vi "demo04_medCal.vi"() -> ()   [LabVIEW 2017]
panel:
  out "过程显示":string
  out "结果":string
  out "输入  2":string
  out "输入  1":string
  out "输入 临时值":string
  out "操作 临时值":string
  in  "操作 等于":bool
  in  "操作 清除":bool
  in  "操作 /":bool
  in  "操作 *":bool
  in  "操作 -":bool
  in  "操作 +":bool
  in  "小数点":bool
  in  "数字 0":bool
  in  "+/-":bool
  in  "数字 9":bool
  in  "数字 8":bool
  in  "数字 7":bool
  in  "数字 6":bool
  in  "数字 5":bool
  in  "数字 4":bool
  in  "数字 3":bool
  in  "数字 2":bool
  in  "数字 1":bool
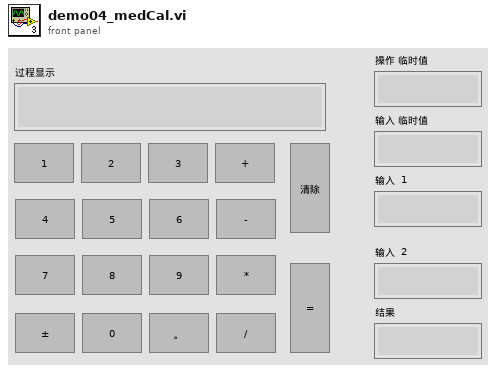
[diagram p1: front panel]
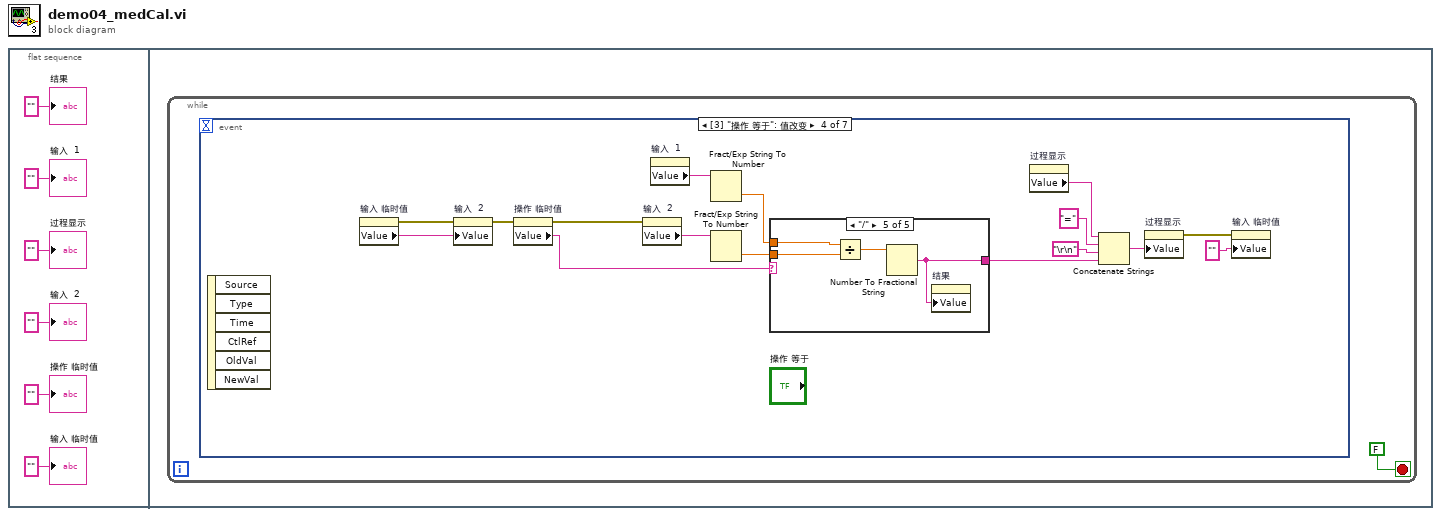
[diagram p0: block diagram]
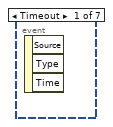
[diagram p2: hidden frame]
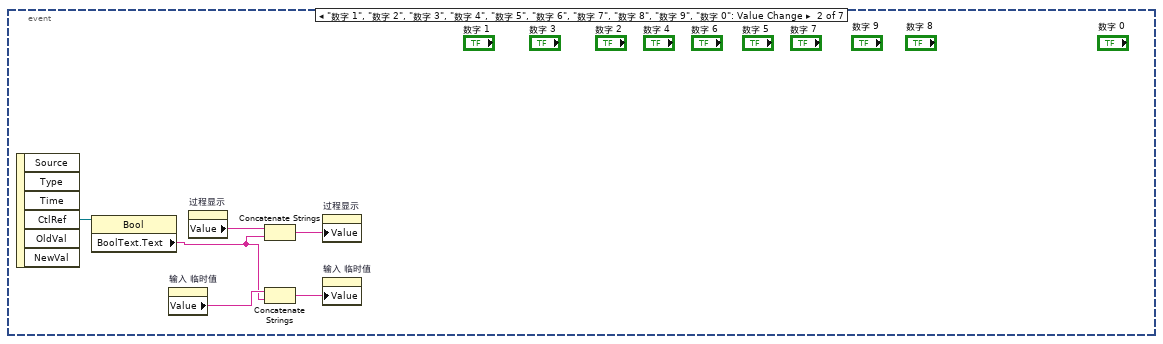
[diagram p3: hidden frame]
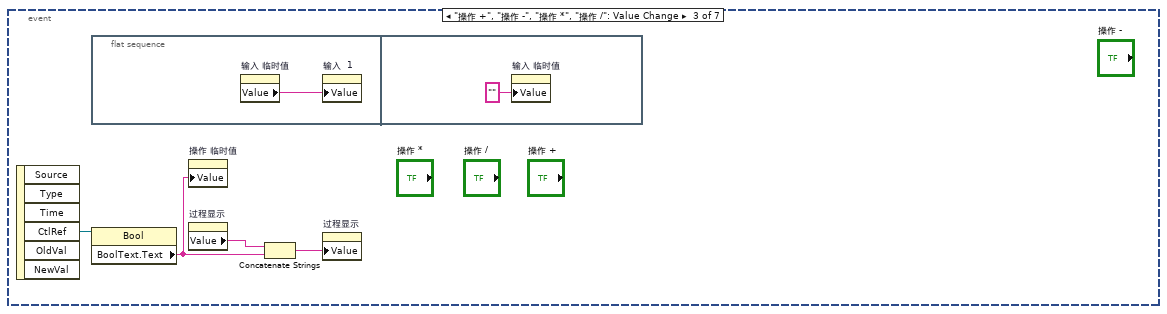
[diagram p4: hidden frame]
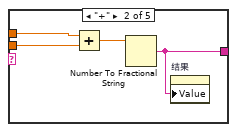
[diagram p6: hidden frame]
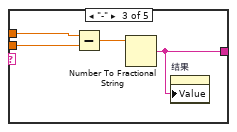
[diagram p7: hidden frame]
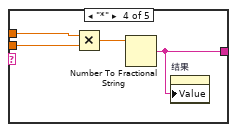
[diagram p8: hidden frame]
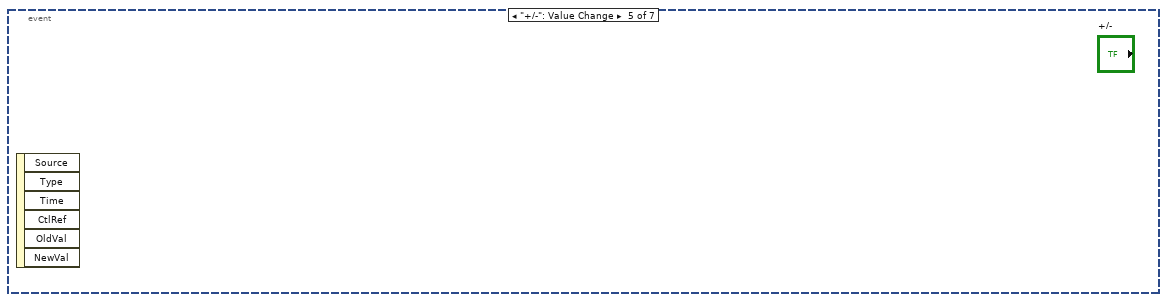
[diagram p9: hidden frame]
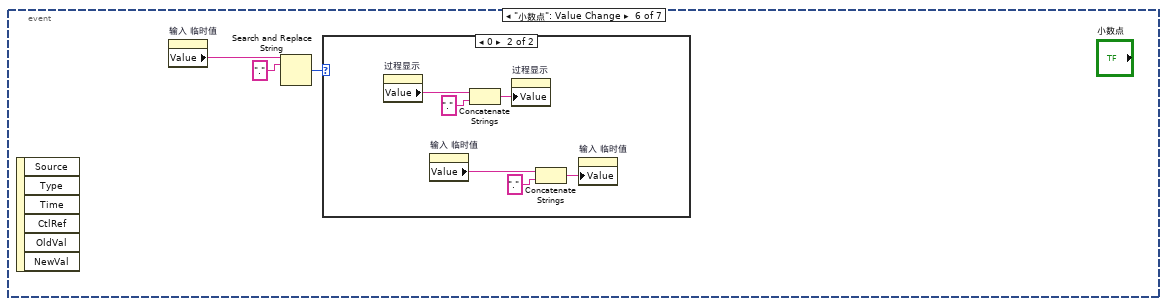
[diagram p10: hidden frame]
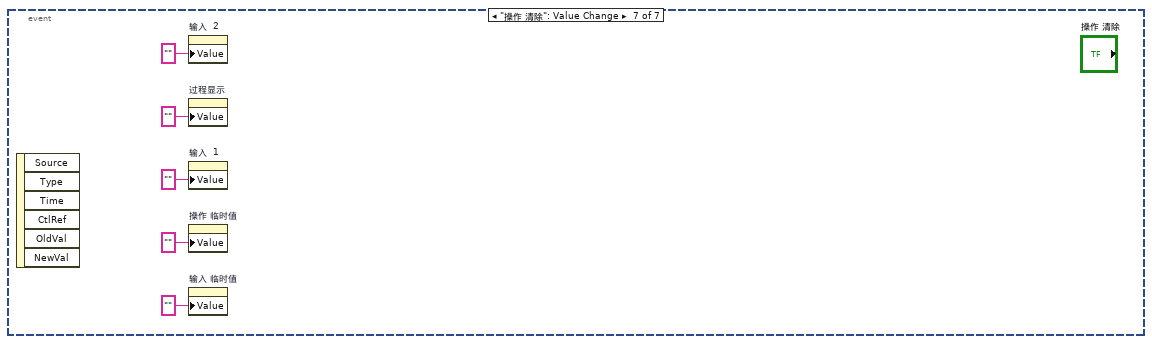
[diagram p12: hidden frame]
diagram:
  n1 = flat-sequence {
    frame #0 {
      "输入 临时值" <- "" ("输入 临时值")
      "输入  1" <- "" ("输入  1")
      "过程显示" <- "" ("过程显示")
      "操作 临时值" <- "" ("操作 临时值")
      "输入  2" <- "" ("输入  2")
      "结果" <- "" ("结果")
    }
    frame #1 {
      n2 = while {
        stop <- FALSE stop-if-true
        n3 = event shown="[3] \"操作 等于\": 值改变" {
          selector: _ -> [_ _ _ _ _ _ _]
          dyn-events: _ -> [_ _ _ _ _ _ _]
          timeout: _ -> [_ _ _ _ _ _ _]
          event Timeout {
            n4 = event-data() -> ()  [unwired: 1 in, 3 out]
          }
          event "数字 1", "数字 2", "数字 3", "数字 4", "数字 5", "数字 6", "数字 7", "数字 8", "数字 9", "数字 0": Value Change {
            n5 = event-data() -> ("CtlRef"=w13:refnum<vi>)  [unwired: 1 in, 5 out]
            n6 = property class="Bool"(reference=w13) -> ("BoolText.Text"=w8:string)  [unwired: 1 in, 2 out]
            n7 = property on="输入 临时值" class="Str"() -> ("Value"=w12:string)  [unwired: 2 in, 2 out]
            n8 = property on="过程显示" class="Str"() -> ("Value"=w9:string)  [unwired: 2 in, 2 out]
            n9 = Concatenate Strings(w9, w8) -> (w10:string)
            n10 = Concatenate Strings(w12, w8) -> (w11:string)
            n11 = property on="过程显示" class="Str"("Value"=w10) -> ()  [unwired: 2 in, 2 out]
            n12 = property on="输入 临时值" class="Str"("Value"=w11) -> ()  [unwired: 2 in, 2 out]
          }
          event "操作 +", "操作 -", "操作 *", "操作 /": Value Change {
            n13 = event-data() -> ("CtlRef"=w17:refnum<vi>)  [unwired: 1 in, 5 out]
            n14 = flat-sequence {
              frame #0 {
                n15 = property on="输入 临时值" class="Str"() -> ("Value"=w18:string)  [unwired: 2 in, 2 out]
                n16 = property on="输入  1" class="Str"("Value"=w18) -> ()  [unwired: 2 in, 2 out]
              }
              frame #1 {
                n17 = property on="输入 临时值" class="Str"("Value"="" ("输入 临时值")) -> ()  [unwired: 2 in, 2 out]
              }
            }
            n18 = property class="Bool"(reference=w17) -> ("BoolText.Text"=w14:string)  [unwired: 1 in, 2 out]
            n19 = property on="操作 临时值" class="Str"("Value"=w14) -> ()  [unwired: 2 in, 2 out]
            n20 = property on="过程显示" class="Str"() -> ("Value"=w15:string)  [unwired: 2 in, 2 out]
            n21 = Concatenate Strings(w15, w14) -> (w16:string)
            n22 = property on="过程显示" class="Str"("Value"=w16) -> ()  [unwired: 2 in, 2 out]
          }
          event "操作 等于": Value Change {
            n23 = event-data() -> ()  [unwired: 1 in, 6 out]
            n24 = property on="输入 临时值" class="Str"() -> (error out=w33:errorcluster, "Value"=w35:string)  [unwired: 2 in, 1 out]
            n25 = property on="输入  2" class="Str"(error in=w33, "Value"=w35) -> (error out=w32:errorcluster)  [unwired: 1 in, 1 out]
            n26 = property on="操作 临时值" class="Str"(error in=w32) -> (error out=w29:errorcluster, "Value"=w34:string)  [unwired: 1 in, 1 out]
            n27 = property on="输入  2" class="Str"(error in=w29) -> ("Value"=w30:string)  [unwired: 1 in, 2 out]
            n28 = property on="输入  1" class="Str"() -> ("Value"=w31:string)  [unwired: 2 in, 2 out]
            n29 = Fract/Exp String To Number(string=w31) -> (number=w28:dbl)  [unwired: 3 in, 1 out]
            n30 = Fract/Exp String To Number(string=w30) -> (number=w27:dbl)  [unwired: 3 in, 1 out]
            n31 = case shown="\"/\"" w34 {
              tunnel: w28 -> [_ w39 w43 w46 w50]
              tunnel: w27 -> [_ w38 w42 w45 w49]
              tunnel: [_ w36 w40 w44 w48] -> w22
              frame "假", Default {
              }
              frame "+" {
                n32 = Add(x=w39, y=w38) -> (x+y=w37:dbl)
                n33 = Number To Fractional String(number=w37) -> (F-format string=w36:string)  [unwired: 3 in]
                n34 = property on="结果" class="Str"("Value"=w36) -> ()  [unwired: 2 in, 2 out]
              }
              frame "-" {
                n35 = Subtract(x=w43, y=w42) -> (x-y=w41:dbl)
                n36 = Number To Fractional String(number=w41) -> (F-format string=w40:string)  [unwired: 3 in]
                n37 = property on="结果" class="Str"("Value"=w40) -> ()  [unwired: 2 in, 2 out]
              }
              frame "*" {
                n38 = Multiply(x=w46, y=w45) -> (x*y=w47:dbl)
                n39 = Number To Fractional String(number=w47) -> (F-format string=w44:string)  [unwired: 3 in]
                n40 = property on="结果" class="Str"("Value"=w44) -> ()  [unwired: 2 in, 2 out]
              }
              frame "/" {
                n41 = Divide(x=w50, y=w49) -> (x/y=w51:dbl)
                n42 = Number To Fractional String(number=w51) -> (F-format string=w48:string)  [unwired: 3 in]
                n43 = property on="结果" class="Str"("Value"=w48) -> ()  [unwired: 2 in, 2 out]
              }
            }
            n44 = property on="过程显示" class="Str"() -> ("Value"=w25:string)  [unwired: 2 in, 2 out]
            n45 = Concatenate Strings(w25, "=" ("字符串"), "\r\n", w22) -> (w26:string)
            n46 = property on="过程显示" class="Str"("Value"=w26) -> (error out=w20:errorcluster)  [unwired: 2 in, 1 out]
            n47 = property on="输入 临时值" class="Str"(error in=w20, "Value"="" ("输入 临时值")) -> ()  [unwired: 1 in, 2 out]
          }
          event "+/-": Value Change {
            n48 = event-data() -> ()  [unwired: 1 in, 6 out]
          }
          event "小数点": Value Change {
            n49 = event-data() -> ()  [unwired: 1 in, 6 out]
            n50 = property on="输入 临时值" class="Str"() -> ("Value"=w54:string)  [unwired: 2 in, 2 out]
            n51 = Search and Replace String(input string=w54, search string="." ("搜索字符串")) -> (number of replacements=w52:i32)  [unwired: 6 in, 3 out]
            n52 = case shown="0" w52 {
              frame 1, Default {
              }
              frame 0 {
                n53 = property on="过程显示" class="Str"() -> ("Value"=w55:string)  [unwired: 2 in, 2 out]
                n54 = property on="输入 临时值" class="Str"() -> ("Value"=w60:string)  [unwired: 2 in, 2 out]
                n55 = Concatenate Strings(w55, "." ("字符串")) -> (w57:string)
                n56 = property on="过程显示" class="Str"("Value"=w57) -> ()  [unwired: 2 in, 2 out]
                n57 = Concatenate Strings(w60, "." ("字符串")) -> (w59:string)
                n58 = property on="输入 临时值" class="Str"("Value"=w59) -> ()  [unwired: 2 in, 2 out]
              }
            }
          }
          event "操作 清除": Value Change {
            n59 = event-data() -> ()  [unwired: 1 in, 6 out]
            n60 = property on="输入  2" class="Str"("Value"="" ("输入  2")) -> ()  [unwired: 2 in, 2 out]
            n61 = property on="过程显示" class="Str"("Value"="" ("过程显示")) -> ()  [unwired: 2 in, 2 out]
            n62 = property on="输入  1" class="Str"("Value"="" ("输入  1")) -> ()  [unwired: 2 in, 2 out]
            n63 = property on="操作 临时值" class="Str"("Value"="" ("操作 临时值")) -> ()  [unwired: 2 in, 2 out]
            n64 = property on="输入 临时值" class="Str"("Value"="" ("输入 临时值")) -> ()  [unwired: 2 in, 2 out]
          }
        }
      }
    }
  }
